vi "Unpack Zip.vi"(8 "error in (no error)":errorcluster, 11 "Zip":path) -> (0 "error out":errorcluster, 2 "Solver VI":path, 3 "Folder":path)   [LabVIEW 2024, in "Wordle Scorer.lvlib"]
uses:
  Wordle Scorer.lvlib
  <vilib>/zip/NI_Unzip.lvlib
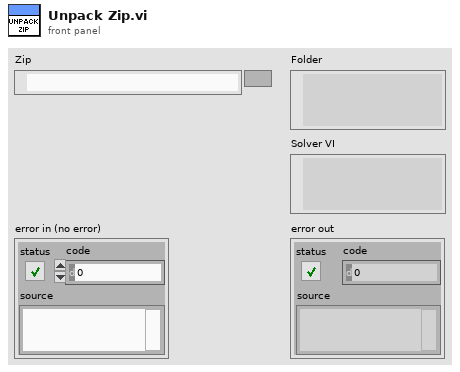
[diagram p1: front panel]
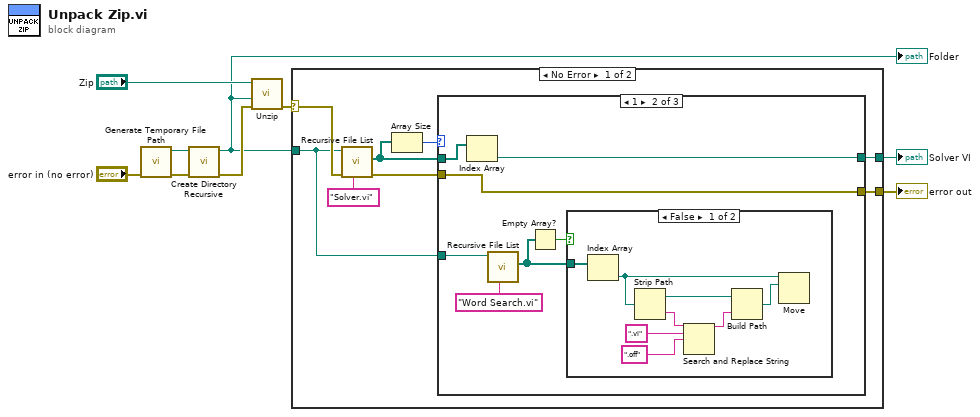
[diagram p0: block diagram]
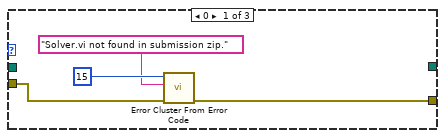
[diagram p2: hidden frame]
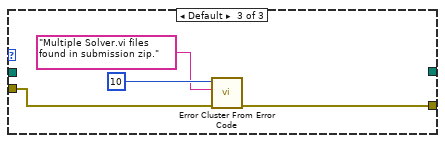
[diagram p4: hidden frame]
diagram:
  n1 = call <vilib>:"Generate Temporary File Path.vi"("error in (no error)"="error in (no error)") -> ("error out"=w6:errorcluster, "Unique Temporary File Path"=w7:path)  [unwired: 9 in]
  n2 = call <vilib>:"Create Directory Recursive.vi"("error in (no error)"=w6, "directory"=w7) -> ("error out"=w5:errorcluster, "directory copy"=w3:path)  [unwired: 3 in, 1 out]
  "Folder" <- w3
  n3 = call <vilib>:"Unzip.vi"("error in (no error)"=w5, "Target directory (same as Zip file if empty)"=w3, "Zip file"="Zip") -> ("error out"=w1:errorcluster)  [unwired: 6 in, 2 out]
  n4 = case shown="No Error" w1 {
    selector: w1 -> [w17 _]
    tunnel: w3 -> [w10 _]
    tunnel: [w12 _] -> w2
    tunnel: [w11 _] -> w9
    frame No Error {
      n5 = call <vilib>:"Recursive File List.vi"("pattern"="Solver.vi", "error in (no error)"=w17, "Folder Path"=w10) -> ("error out"=w13:errorcluster, "All Files in Dir"=w14:path[])  [unwired: 4 in, 3 out]
      n6 = Array Size(array=w14) -> (size(s)=w15:i32)
      n7 = case shown="1" w15 {
        tunnel: w14 -> [_ w28 _]
        tunnel: w13 -> [w21 w26 w39]
        tunnel: [_ w27 _] -> w12
        tunnel: [w18 w26 w40] -> w11
        tunnel: w10 -> [_ w25 _]
        frame 0 {
          n8 = call <vilib>:"Error Cluster From Error Code.vi"("error in (no error)"=w21, "error message (\"\")"="Solver.vi not found in submission zip.", "error code (0)"=15) -> ("error out"=w18:errorcluster)  [unwired: 6 in]
        }
        frame 1 {
          n9 = Index Array(array=w28) -> (element=w27:path)  [unwired: 1 in]
          n10 = call <vilib>:"Recursive File List.vi"("pattern"="Word Search.vi", "Folder Path"=w25) -> ("All Files in Dir"=w23:path[])  [unwired: 5 in, 4 out]
          n11 = Empty Array?(array=w23) -> (empty?=w22:bool)
          n12 = case shown="False" w22 {
            tunnel: w23 -> [w36 _]
            frame False {
              n13 = Index Array(array=w36) -> (element=w35:path)  [unwired: 1 in]
              n14 = Strip Path(path=w35) -> (stripped path=w31:path, name=w34:string)
              n15 = Search and Replace String(input string=w34, search string=".vi", replace string=".off" ("search string")) -> (result string=w30:string)  [unwired: 5 in, 3 out]
              n16 = Build Path(base path=w31, name or relative path=w30) -> (appended path=w29:path)
              n17 = Move(source path=w35, 10:w29) -> ()  [unwired: 3 in, 3 out]
            }
            frame True {
            }
          }
        }
        frame Default {
          n18 = call <vilib>:"Error Cluster From Error Code.vi"("error in (no error)"=w39, "error message (\"\")"="Multiple Solver.vi files found in submission zip.", "error code (0)"=10) -> ("error out"=w40:errorcluster)  [unwired: 6 in]
        }
      }
    }
    frame Error {
    }
  }
  "error out" <- w9
  "Solver VI" <- w2
